vi "Tune.vi"(11 "Tune":bool=TRUE) -> ()   [LabVIEW 2025, in "Controls.lvlib"]
uses:
  Controls.lvlib
  Global 2.vi
panel:
  in  "Wideband":bool
  in  "Done":bool
  in  "Phase Voltage":dbl=2.566 format="%_4g"
  in  "Tune Voltage":dbl=1.8849999999999991 min=0.0 max=8.0 format="%_5g"
  in  "Mode":T1(ring)
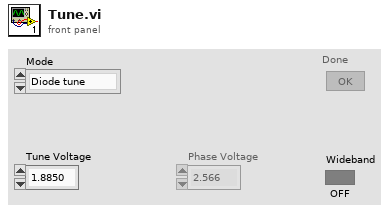
[diagram p1: front panel]
types:
  T1 = enum16{"Diode tune", "Phase tune", "Operating tune"}
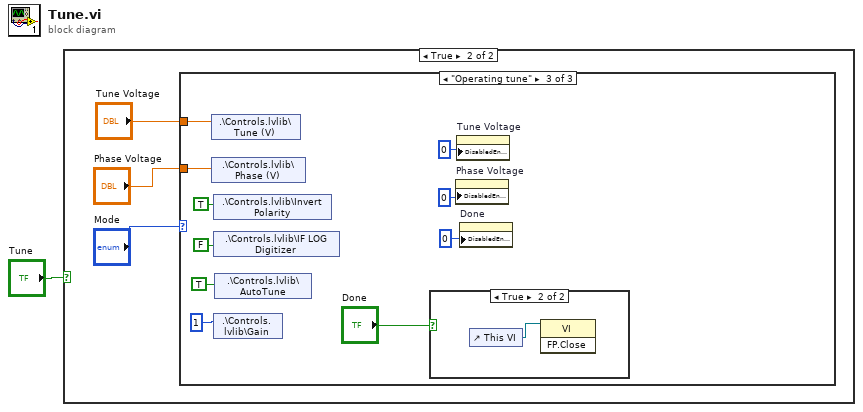
[diagram p0: block diagram]
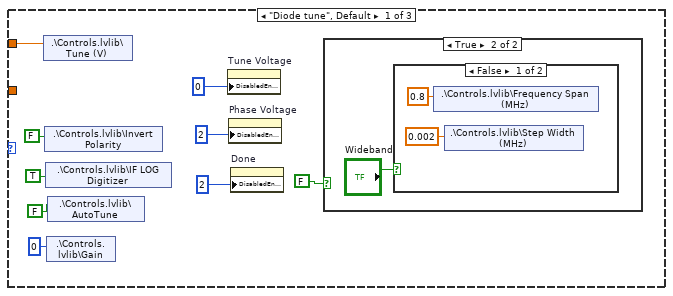
[diagram p3: hidden frame]
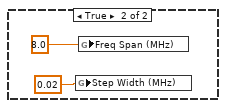
[diagram p5: hidden frame]
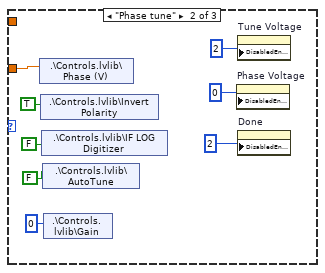
[diagram p6: hidden frame]
diagram:
  n1 = case shown="True" "Tune" {
    frame False {
    }
    frame True {
      n2 = case shown="\"Operating tune\"" "Mode" {
        tunnel: "Tune Voltage" -> [w5 _ w27]
        tunnel: "Phase Voltage" -> [_ w19 w28]
        frame "Diode tune", Default {
          n3 = shared-variable ".\\Controls.lvlib\\Tune (V)"(w5) -> ()  [unwired: 1 in, 1 out]
          n4 = shared-variable ".\\Controls.lvlib\\Invert Polarity"(FALSE) -> ()  [unwired: 1 in, 1 out]
          n5 = shared-variable ".\\Controls.lvlib\\IF LOG Digitizer"(TRUE) -> ()  [unwired: 1 in, 1 out]
          n6 = shared-variable ".\\Controls.lvlib\\Gain"(0) -> ()  [unwired: 1 in, 1 out]
          n7 = shared-variable ".\\Controls.lvlib\\AutoTune"(FALSE) -> ()  [unwired: 1 in, 1 out]
          n8 = property on="Tune Voltage" class="DigNum (strict)"("DisabledEnum"=0) -> ()  [unwired: 2 in, 2 out]
          n9 = property on="Phase Voltage" class="DigNum (strict)"("DisabledEnum"=2) -> ()  [unwired: 2 in, 2 out]
          n10 = property on="Done" class="Bool (strict)"("DisabledEnum"=2) -> ()  [unwired: 2 in, 2 out]
          n11 = case shown="True" FALSE {
            frame False {
            }
            frame True {
              n12 = case shown="False" "Wideband" {
                frame False {
                  n13 = shared-variable ".\\Controls.lvlib\\Frequency Span (MHz)"(0.8) -> ()  [unwired: 1 in, 1 out]
                  n14 = shared-variable ".\\Controls.lvlib\\Step Width (MHz)"(0.002) -> ()  [unwired: 1 in, 1 out]
                }
                frame True {
                  n15 = global write "Global 2.vi" "Step Width (MHz)"(0.02) -> ()
                  n16 = global write "Global 2.vi" "Freq Span (MHz)"(8.0) -> ()
                }
              }
            }
          }
        }
        frame "Phase tune" {
          n17 = shared-variable ".\\Controls.lvlib\\Phase (V)"(w19) -> ()  [unwired: 1 in, 1 out]
          n18 = shared-variable ".\\Controls.lvlib\\Invert Polarity"(TRUE) -> ()  [unwired: 1 in, 1 out]
          n19 = shared-variable ".\\Controls.lvlib\\IF LOG Digitizer"(FALSE) -> ()  [unwired: 1 in, 1 out]
          n20 = shared-variable ".\\Controls.lvlib\\AutoTune"(FALSE) -> ()  [unwired: 1 in, 1 out]
          n21 = shared-variable ".\\Controls.lvlib\\Gain"(0) -> ()  [unwired: 1 in, 1 out]
          n22 = property on="Phase Voltage" class="DigNum (strict)"("DisabledEnum"=0) -> ()  [unwired: 2 in, 2 out]
          n23 = property on="Tune Voltage" class="DigNum (strict)"("DisabledEnum"=2) -> ()  [unwired: 2 in, 2 out]
          n24 = property on="Done" class="Bool (strict)"("DisabledEnum"=2) -> ()  [unwired: 2 in, 2 out]
        }
        frame "Operating tune" {
          n25 = shared-variable ".\\Controls.lvlib\\Tune (V)"(w27) -> ()  [unwired: 1 in, 1 out]
          n26 = shared-variable ".\\Controls.lvlib\\Phase (V)"(w28) -> ()  [unwired: 1 in, 1 out]
          n27 = shared-variable ".\\Controls.lvlib\\Invert Polarity"(TRUE) -> ()  [unwired: 1 in, 1 out]
          n28 = shared-variable ".\\Controls.lvlib\\IF LOG Digitizer"(FALSE) -> ()  [unwired: 1 in, 1 out]
          n29 = shared-variable ".\\Controls.lvlib\\Gain"(1) -> ()  [unwired: 1 in, 1 out]
          n30 = shared-variable ".\\Controls.lvlib\\AutoTune"(TRUE) -> ()  [unwired: 1 in, 1 out]
          n31 = case shown="True" "Done" {
            frame False {
            }
            frame True {
              n32 = control-ref of="This VI"() -> (w37:refnum<vi>)
              n33 = invoke class="VI" method="FP.Close"(reference=w37) -> ()  [unwired: 2 in, 3 out]
            }
          }
          n34 = property on="Phase Voltage" class="DigNum (strict)"("DisabledEnum"=0) -> ()  [unwired: 2 in, 2 out]
          n35 = property on="Tune Voltage" class="DigNum (strict)"("DisabledEnum"=0) -> ()  [unwired: 2 in, 2 out]
          n36 = property on="Done" class="Bool (strict)"("DisabledEnum"=0) -> ()  [unwired: 2 in, 2 out]
        }
      }
    }
  }
